vi "CS++ExampleContent.vi"() -> (0 "CS++Classes & Messages":T1(array[cluster]))   [LabVIEW 2014]
doc: "Place actor and class constants that should be included included in an application on the blockdiagramm."
uses:
  <vilib>/ActorFramework/Message/Message.lvclass
  Classes/Example/Example.lvclass
  Actors/PVClient-Example/PVClient-Example.lvclass
  CSPP_Core/Actors/CS++BaseActor/CS++BaseActor.lvclass
panel:
  # "Place actor and class constants on the blockdiagramm."
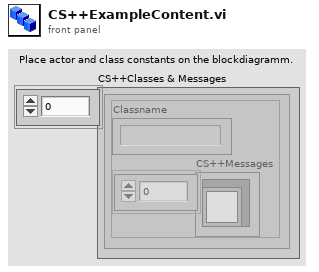
[diagram p1: front panel]
types:
  T1 = cluster{"Classname":string, "CS++Messages":refnum<class "Message.lvclass">[]}[]
  T2 = cluster{"class name":string, "CS++Messages":refnum<class "Message.lvclass">[]}
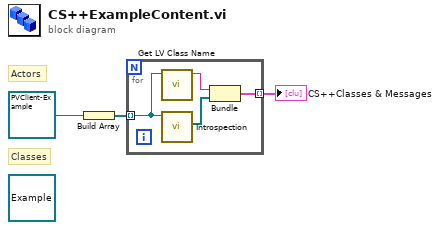
[diagram p0: block diagram]
diagram:
  (unwired) refnum<class "Example.lvclass"> refnum ("CS++Core-Examples.lvlib:Example.lvclass")
  # "Classes"
  # "Actors"
  n1 = Build Array(refnum<class "PVClient-Example.lvclass"> refnum ("PVClient-Example.lvlib:PVClient-Example.lvclass")) -> (w3:refnum<class "PVClient-Example.lvclass">[])
  n2 = for {
    tunnel: w3 -> [w7] mode=indexing
    tunnel: [w4] -> w2 mode=indexing
    n3 = call <vilib>:"Get LV Class Name.vi"("object"=w7) -> ("class name"=w6:string)  [unwired: 9 in, 1 out]
    n4 = call "Introspection.vi"("CS++BaseActor in"=w7) -> ("CS++Messages"=w5:refnum<class "Message.lvclass">[])  [unwired: 8 in, 2 out]
    n5 = Bundle("class name"=w6, "CS++Messages"=w5) -> (w4:T2)  [unwired: 1 in]
  }
  "CS++Classes & Messages" <- w2
